vi "Calculate.vi"(8 "error in (no error)":errorcluster, 10 "X (degrees)":dbl, 11 "AngleFunction in":refnum<class "AbstractAngleFunction.lvclass">) -> (0 "error out":errorcluster, 2 "AngleFunction(X)":dbl, 3 "AngleFunction out":refnum<class "AbstractAngleFunction.lvclass">)   [LabVIEW 2013, in "AbstractAngleFunction.lvclass"]
uses:
  AbstractAngleFunction.lvclass
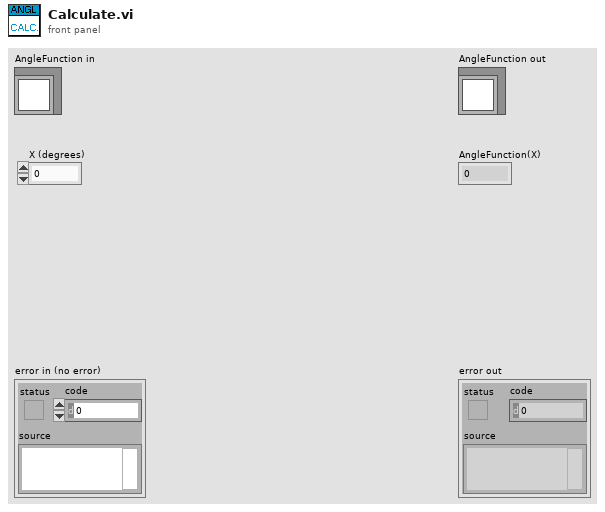
[diagram p1: front panel]
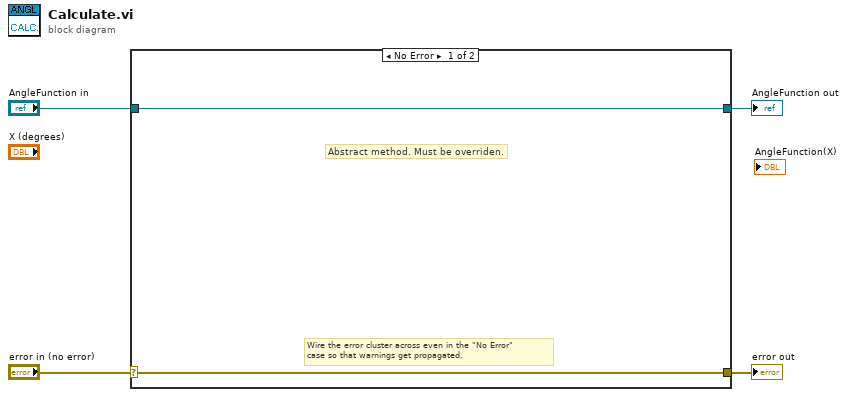
[diagram p0: block diagram]
diagram:
  n1 = case shown="No Error" "error in (no error)" {
    selector: "error in (no error)" -> [w5 w8]
    tunnel: [w5 w8] -> w3
    tunnel: [w6 w7] -> w1
    tunnel: "AngleFunction in" -> [w6 w7]
    frame No Error {
      # "Abstract method. Must be overriden."
      # "Wire the error cluster across even in the \"No Error\"\ncase so that warnings get propagated."
    }
    frame Error {
    }
  }
  "error out" <- w3
  "AngleFunction out" <- w1
